vi "Get Status Channels references.vi"(8 "error in (no error)":errorcluster, 10 "Page":string, 11 "Device Reference in":T4 format="%.0x") -> (0 "error out":errorcluster, 2 "Status Ref":T3 {"Block Data Refs"."Data Reference" format="%.0x"}, 3 "Device Reference out":T4=18446744073709551615 format="%.0x")   [LabVIEW 2020, in "Shared Variables CD 2.0 Engine.lvlib"]
uses:
  Shared Variables CD 2.0 Engine.lvlib
  <vilib>/NI VeriStand/Custom Device API/Custom Device Item Ref.ctl
  <vilib>/NI VeriStand/Custom Device API/Block Data Reference.ctl
  <vilib>/NI VeriStand/Custom Device API/Data Reference.ctl
  <vilib>/NI VeriStand/Custom Device API/Data Access Type.ctl
  <vilib>/Utility/error.llb/Error Cluster From Error Code.vi
  <vilib>/ErrorRing/Error Ring.xnode
  <vilib>/NI VeriStand/Custom Device Tools/Custom Device Utility Library/Custom Device Utility Library.lvlib
  <vilib>/NI VeriStand/Custom Device API/Custom Device API.lvlib
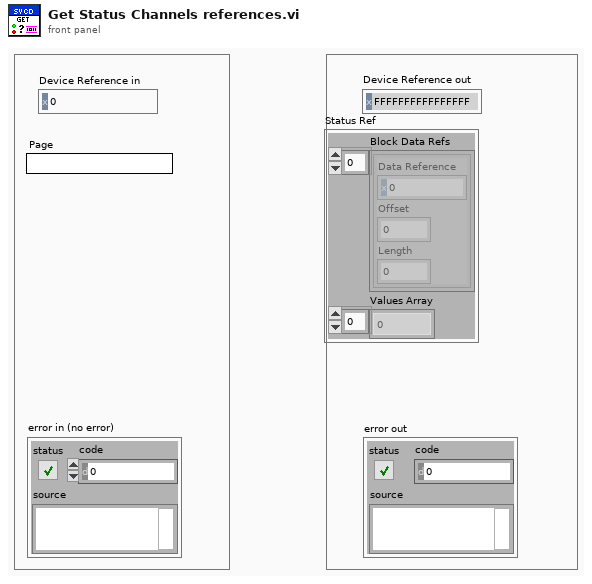
[diagram p1: front panel]
types:
  T1 = typedef "Custom Device API.lvlib/Block Data Reference.ctl" = cluster{"Data Reference":T2, "Offset":u64, "Length":u64}
  T2 = typedef "Custom Device API.lvlib/Data Reference.ctl" = i32
  T3 = cluster{"Block Data Refs":T1[], "Values Array":dbl[]}
  T4 = typedef "Custom Device API.lvlib/Custom Device Item Ref.ctl" = u64
  T5 = typedef "Custom Device API.lvlib/Data Access Type.ctl" = enum16{"Read", "Write"}
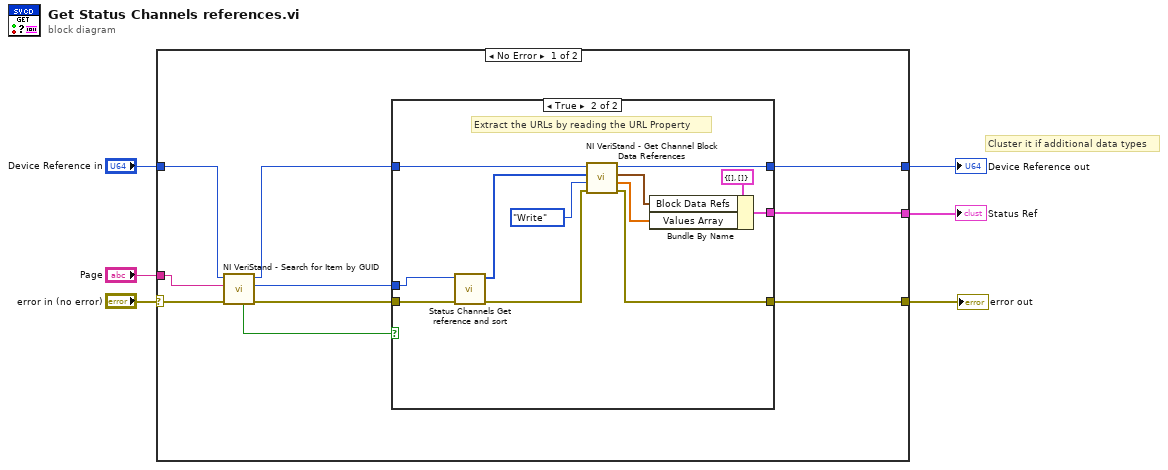
[diagram p0: block diagram]
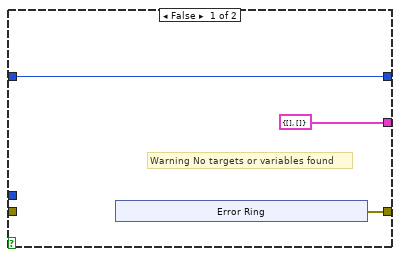
[diagram p2: hidden frame]
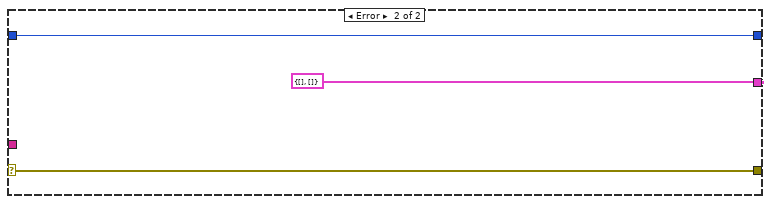
[diagram p3: hidden frame]
diagram:
  # "Cluster it if additional data types"
  n1 = case shown="No Error" "error in (no error)" {
    selector: "error in (no error)" -> [w13 w38]
    tunnel: [w16 w38] -> w6
    tunnel: "Device Reference in" -> [w15 w39]
    tunnel: "Page" -> [w14 _]
    tunnel: [w8 w39] -> w3
    tunnel: [w7 T3 {"Block Data Refs"=[], "Values Array"=[]} ("Status Ref")] -> w1
    frame No Error {
      n2 = call <vilib>:"NI VeriStand - Search for Item by GUID.vi"("error in"=w13, "Item GUID"=w14, "Section Ref in"=w15) -> ("error out"=w11:errorcluster, "Item Ref"=w10:T4, "Section Ref out"=w9:T4, "Found"=w12:bool)  [unwired: 5 in]
      n3 = case shown="True" w12 {
        tunnel: [w19 w33] -> w16
        tunnel: w11 -> [_ w35]
        tunnel: w10 -> [_ w36]
        tunnel: w9 -> [w18 w31]
        tunnel: [w18 w29] -> w8
        tunnel: [T3 {"Block Data Refs"=[], "Values Array"=[]} ("Status Ref") w27] -> w7
        frame False {
          # "Warning No targets or variables found"
          n4 = xnode "Error Ring"() -> ("error out"=w19:errorcluster)
        }
        frame True {
          # "Extract the URLs by reading the URL Property"
          n5 = call "Status Channels Get reference and sort.vi"("error in (no error)"=w35, "Item Ref"=w36) -> ("error out"=w34:errorcluster, "Channel Refs"=w32:T4[])  [unwired: 8 in]
          n6 = call <vilib>:"NI VeriStand - Get Channel Block Data References.vi"("error in (no error)"=w34, "Access"=Data_Access_Type."Write", "Channel Refs"=w32, "Device Ref in"=w31) -> ("error out"=w33:errorcluster, "Values Array"=w25:dbl[], "Block Data Refs"=w26:T1[], "Device Ref out"=w29:T4)  [unwired: 4 in]
          n7 = Bundle By Name(cluster=T3 {"Block Data Refs"=[], "Values Array"=[]} ("Status Ref"), "Block Data Refs"=w26, "Values Array"=w25) -> (w27:T3)
        }
      }
    }
    frame Error {
    }
  }
  "error out" <- w6
  "Device Reference out" <- w3
  "Status Ref" <- w1
